vi "RndBeamF.vi"(1 "size (default 128)":i32=128, 2 "重复次数":i32=20) -> (0 "数组":cdb[][](array[numeric]))   [LabVIEW 2018]
panel:
  out "强度图 3":dbl[][](graph)
  out "强度图 2":dbl[][](graph)
  out "强度图":dbl[][](graph)
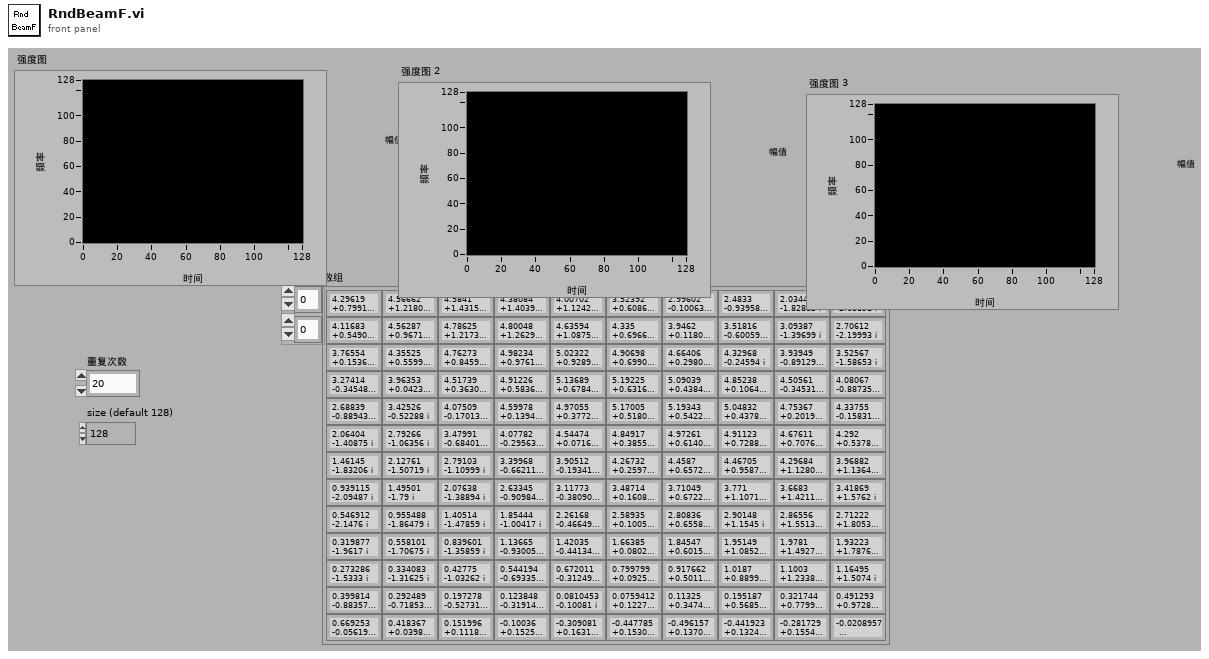
[diagram p1: front panel]
types:
  T1 = cluster{"amplitude matrix":cdb[][], "number of columns in amplitude matrix":i32, "number of rows in amplitude matrix":i32, "represented width (in m)":dbl, "represented height (in m)":dbl, "wavelength (in m)":dbl}
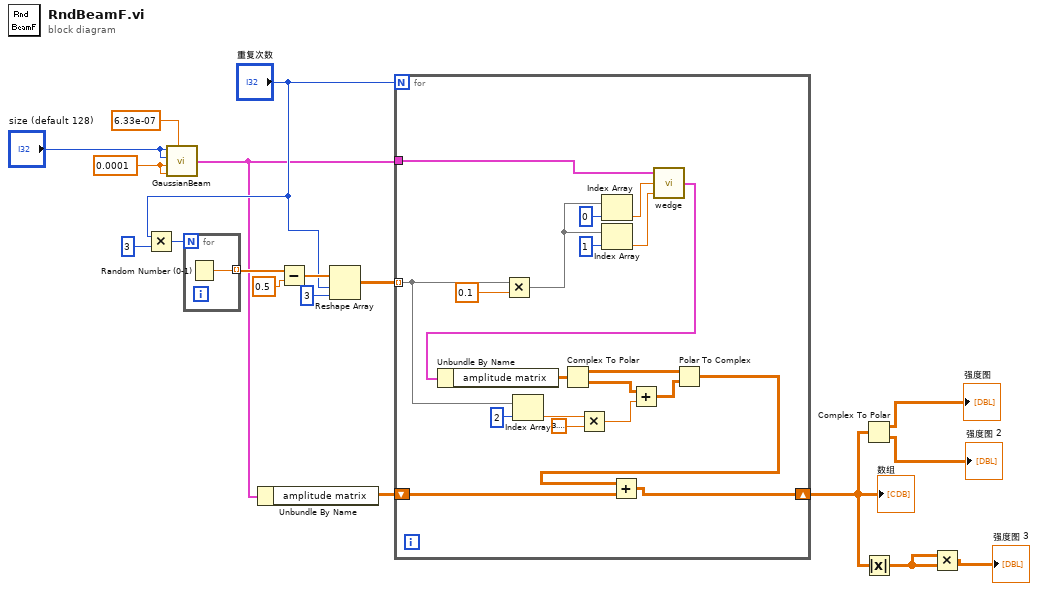
[diagram p0: block diagram]
diagram:
  w17 = 0.0001 ("width of represented x range (in m; default 1E-3=1mm)")
  n1 = Multiply(x="重复次数", y=3) -> (x*y=w15:i32)
  n2 = call "GaussianBeam.vi"("wavelength (in m; default 633E-9=633nm)"=6.33e-07, "width of represented y range (in m; default 1E-3=1mm)"=w17, "width of represented x range (in m; default 1E-3=1mm)"=w17, "number of rows in amplitude matrix (default 64)"="size (default 128)", "number of columns in amplitude matrix (default 64)"="size (default 128)") -> ("Gaussian beam"=w7:T1)  [unwired: 1 in]
  n3 = for {
    N: w15 -> [_]
    tunnel: [w19] -> w13 mode=indexing
    n4 = Random Number (0-1)() -> (number: 0 to 1=w19:dbl)
  }
  n5 = Unbundle By Name(w7) -> ("amplitude matrix"=w6:cdb[][])
  n6 = Subtract(x=w13, y=0.5) -> (x-y=w11:dbl[])
  n7 = Reshape Array(w11, "重复次数", 3 ("维数大小")) -> (w8:dbl[][])
  n8 = for {
    N: "重复次数" -> [_]
    tunnel: w7 -> [w30]
    shift-right: [w39] -> w5
    shift-left: w6 -> [w38]
    tunnel: w8 -> [w25] mode=indexing
    n9 = Multiply(x=w25, y=0.1) -> (x*y=w35:dbl[])
    n10 = Index Array(array=w25, index=2 ("索引")) -> (element=w24:dbl)
    n11 = Multiply(x=w24, y=3.141592653589793) -> (x*y=w20:dbl)
    n12 = Index Array(array=w35, index=0 ("索引")) -> (element=w32:dbl)
    n13 = Index Array(array=w35, index=1 ("索引")) -> (element=w31:dbl)
    n14 = call "wedge.vi"("angle in y-z plane, beta"=w31, "angle in x-z plane, alpha"=w32, "beam in front of spiral wave plate"=w30) -> ("beam behind spiral wave plate"=w37:T1)
    n15 = Unbundle By Name(w37) -> ("amplitude matrix"=w29:cdb[][])
    n16 = Complex To Polar(r * e^(i*theta)=w29) -> (r=w28:dbl[][], theta=w21:dbl[][])
    n17 = Add(x=w21, y=w20) -> (x+y=w22:dbl[][])
    n18 = Polar To Complex(1:w22, 2:w28) -> (0:w27:cdb[][])
    n19 = Add(x=w27, y=w38) -> (x+y=w39:cdb[][])
  }
  "数组" <- w5
  n20 = Complex To Polar(r * e^(i*theta)=w5) -> (r=→"强度图":dbl[][], theta=→"强度图 2":dbl[][])
  n21 = Absolute Value(x=w5) -> (abs(x)=w4:dbl[][])
  n22 = Multiply(x=w4, y=w4) -> (x*y=→"强度图 3":dbl[][])
